vi "Open_Top_Level_VIs.vi"(8 "error in (no error)":errorcluster, 11 "Build in":refnum<class "AB_SourceDistribution.lvclass">) -> (0 "error out":errorcluster, 2 "Top-Level VIs":refnum<vi>[](array[refnum]), 3 "Build out":refnum<class "AB_SourceDistribution.lvclass">)   [LabVIEW 2020, in "AB_SourceDistribution.lvclass"]
uses:
  <vilib>/AppBuilder/AB_Classes/SourceDistribution/AB_SourceDistribution.lvclass
  e:/builds/penguin/labview/branches/2020/dev/dist/vi.lib/AppBuilder/AB_Classes/Build/AB_Build.lvclass
  <vilib>/AppBuilder/AB_Classes/Build/AB_Build.lvclass
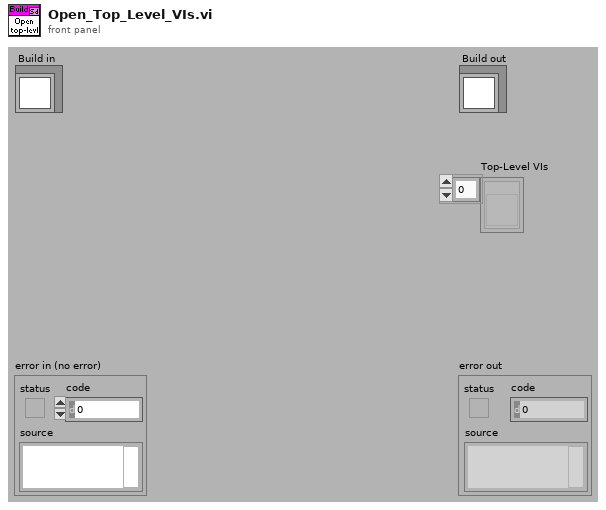
[diagram p1: front panel]
types:
  T1 = typedef "AB_Build.ctl" = cluster{"buildSpecName":string, "buildSpecDescription":string, "destinations":refnum<class "AB_Destination.lvclass">[], "exclusionOption":T2, "defaultLanguage":string, "supportedLanguages":string[], "excludedDirectories":path[], "buildContext":refnum<vi>, "buildObject":T3, "preview":bool, "programatic":bool, "progressBarEvents":T4, "userLog_Path":path, "preActionID":string, "preAction_Path":path, "postActionID":string, "postAction_Path":path, "eng_checkForBrokenVIs?":bool, "eng_verboseLinkerErrors?":bool, "localDest_Path":path, "targetDest_Path":path, "removeVIObject":u16, "cache":refnum<class "PreviewCache.lvclass">, "use cache":bool, "previewCache_ID":string, "buildCache_ID":string, "eng_TempLocalDest_Path":path, "eng_collectDependencies?":bool, "versionInfo":cluster{"buildVersion":cluster{"major":u16, "minor":u16, "patch":u16, "build":u16}, "autoIncrement":bool}, "eng_enableVIChecksums":bool}
  T2 = typedef "AB_Exclusion_Option.ctl" = cluster{"typedefs":bool, "polymorphicVIs":bool, "unusedLibraryItems":bool, "modifyLibraryFile":bool, "edit-timeDependencies":bool, "inlineVIs":bool, "dependent PPLs":bool, "dependent DLLs":bool}
  T3 = typedef "ItemRef.ctl" = u64
  T4 = typedef "provcom_ProgressBar_Events.ctl" = cluster{"newJob":refnum<user-event>, "newItem":refnum<user-event>, "errorMsg":T5, "cancel":refnum<user-event>}
  T5 = typedef "mxLvBuildError.ctl" = refnum<user-event>
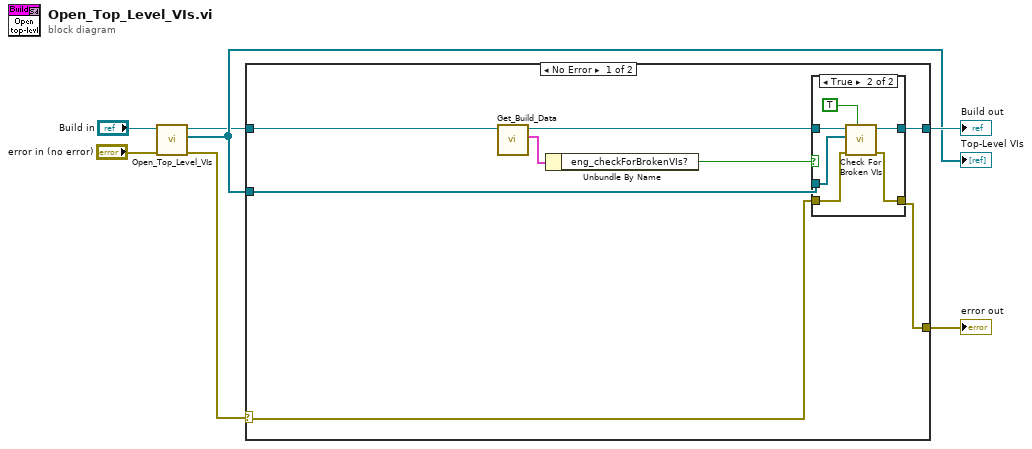
[diagram p0: block diagram]
diagram:
  n1 = call-parent "Open_Top_Level_VIs.vi"("error in (no error)"="error in (no error)", "Build in"="Build in") -> ("error out"=w6:errorcluster, "Top-Level VIs"=w2:refnum<vi>[], "Build out"=w1:refnum<class "AB_SourceDistribution.lvclass">)  [unwired: 7 in]
  "Top-Level VIs" <- w2
  n2 = case shown="No Error" w6 {
    selector: w6 -> [w15 w25]
    tunnel: [w14 w25] -> w5
    tunnel: w2 -> [w8 _]
    tunnel: w1 -> [w13 w24]
    tunnel: [w10 w24] -> w3
    frame No Error {
      n3 = call <vilib>:"Get_Build_Data.vi"("Class in"=w13) -> ("data"=w12:T1, "Class out"=w9:refnum<class "AB_SourceDistribution.lvclass">)  [unwired: 8 in, 1 out]
      n4 = Unbundle By Name(w12) -> ("eng_checkForBrokenVIs?"=w11:bool)
      n5 = case shown="True" w11 {
        tunnel: w8 -> [_ w19]
        tunnel: w15 -> [w16 w20]
        tunnel: [w16 w21] -> w14
        tunnel: [w17 w22] -> w10
        tunnel: w9 -> [w17 w23]
        frame False {
        }
        frame True {
          n6 = call <vilib>:"Check For Broken VIs.vi"("before build?"=TRUE, "error in (no error)"=w20, "Top-Level VIs"=w19, "Class in"=w23) -> ("error out"=w21:errorcluster, "Class out"=w22:refnum<class "AB_SourceDistribution.lvclass">)  [unwired: 6 in]
        }
      }
    }
    frame Error {
    }
  }
  "error out" <- w5
  "Build out" <- w3
